vi "Start Module.vi"(7 "CfgManager":refnum<class "ConfigManager.lvclass">, 8 "error in (no error)":errorcluster, 9 "Owner":refnum<class "UniqueName.lvclass">, 10 "Module Name (empty: default)":string, 11 "Run as Singleton? (F)":bool) -> (0 "error out":errorcluster, 1 "Wait for Event Sync?":bool, 2 "Configurable Broadcast Events":T1, 3 "Module ID":i32)   [LabVIEW 2014, in "Configurable.lvlib"]
doc: "Launches the Module Main.vi.\n_____\nBased on Delacor QMH Project Template 4.0.0.47."
uses:
  Configurable.lvlib
  Broadcast Events--cluster.ctl
  Did Init Argument--cluster.ctl
  Status Updated Argument--cluster.ctl
  Error Reported Argument--cluster.ctl
  Stop Argument--cluster.ctl
  Get Module Execution Status Argument--cluster.ctl
  Module Configuration Argument--cluster.ctl
  ModuleConfiguration--Cluster.ctl
  <vilib>/LabVIEW Open Source/Configuration Manager/Manager/ConfigManager.lvclass
  <vilib>/LabVIEW Open Source Project/Unicity/UniqueName/UniqueNameClass/UniqueName.lvclass
  Module Running State--enum.ctl
  <vilib>/Delacor/Delacor QMH/Libraries/Cloneable Module Admin_class/Delacor_lib_QMH_Cloneable Module Admin.lvclass
  <vilib>/Delacor/Delacor QMH/Libraries/Cloneable Module Admin_class/Delacor_lib_QMH_Cloneable Module Admin.lvclass/Delacor_lib_QMH_Cloneable Module Admin.ctl
  <vilib>/Delacor/Delacor QMH/Libraries/Module Admin_class/Delacor_lib_QMH_Module Admin.lvclass/Delacor_lib_QMH_Module Admin.ctl
  <vilib>/Delacor/Delacor QMH/Libraries/Cloneable Module Admin_class/Delacor_lib_QMH_Set Module ID.vi
  <vilib>/Delacor/Delacor QMH/Libraries/Module Admin_class/Delacor_lib_QMH_Set External Launch.vi
  <vilib>/Utility/error.llb/Error Cluster From Error Code.vi
  <vilib>/ErrorRing/Error Ring.xnode
  Clone Registration/Clone Registration.lvlib
  <vilib>/LabVIEW Open Source/Configuration Manager/Cache/ConfigManager.Cache.lvclass
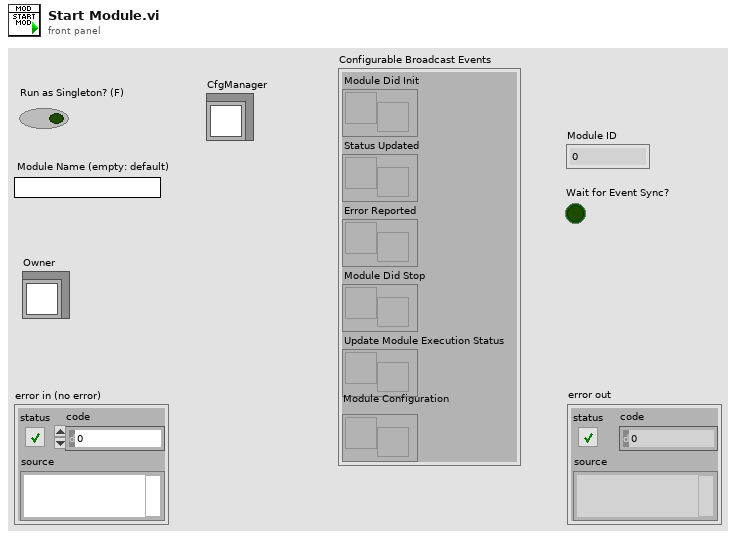
[diagram p1: front panel]
types:
  T1 = typedef "Configurable.lvlib/Broadcast Events--cluster.ctl" = cluster{"Module Did Init":refnum<user-event>, "Status Updated":refnum<user-event>, "Error Reported":refnum<user-event>, "Module Did Stop":refnum<user-event>, "Update Module Execution Status":refnum<user-event>, "Module Configuration":refnum<user-event>}
  T2 = typedef "Configurable.lvlib/Module Running State--enum.ctl" = enum16{"Not Running", "Running as Cloneable", "Running as Singleton"}
  T3 = enum32{"Bad", "Idle", "Run top level", "Running"}
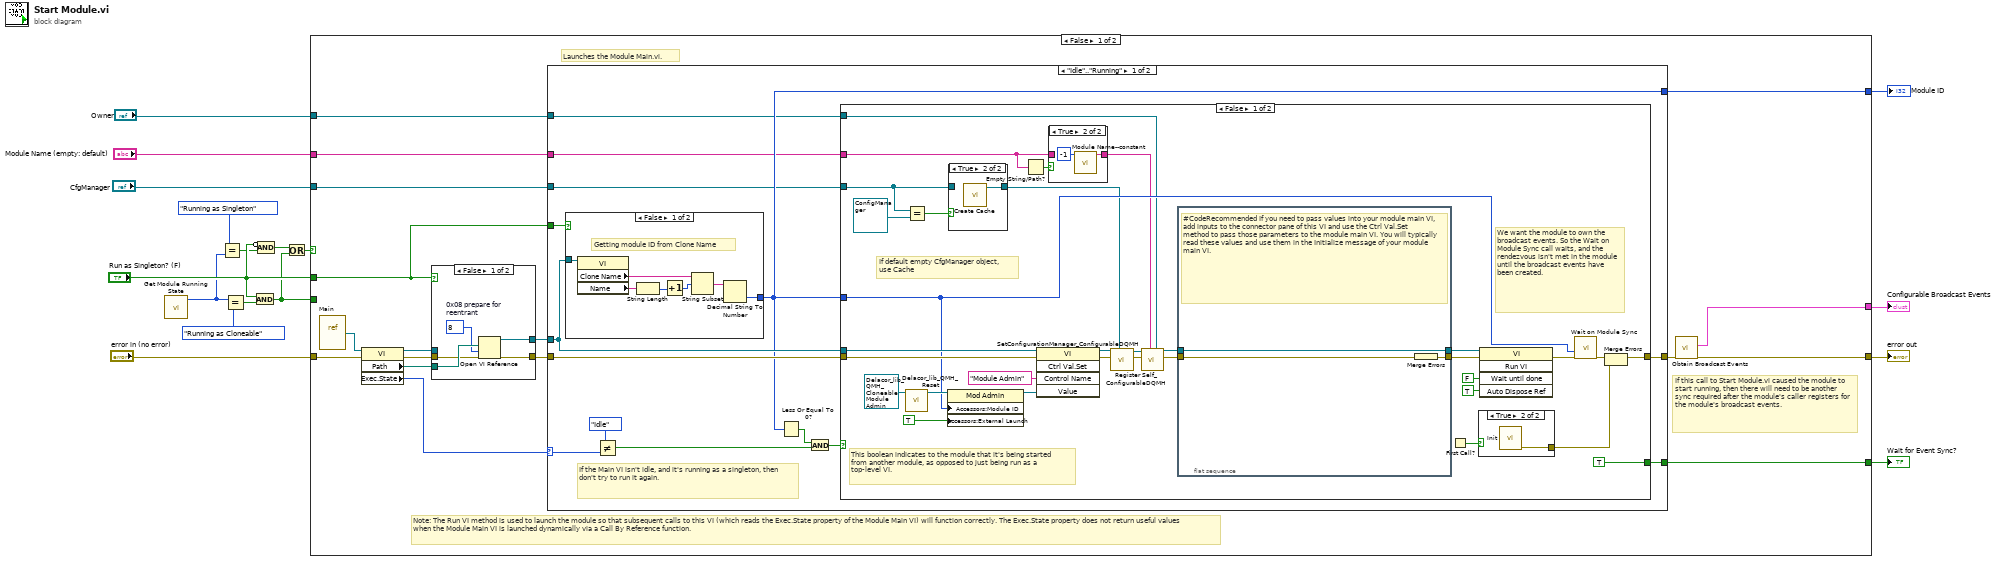
[diagram p0: block diagram]
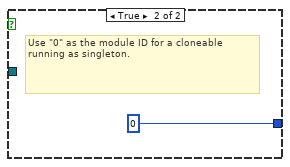
[diagram p3: hidden frame]
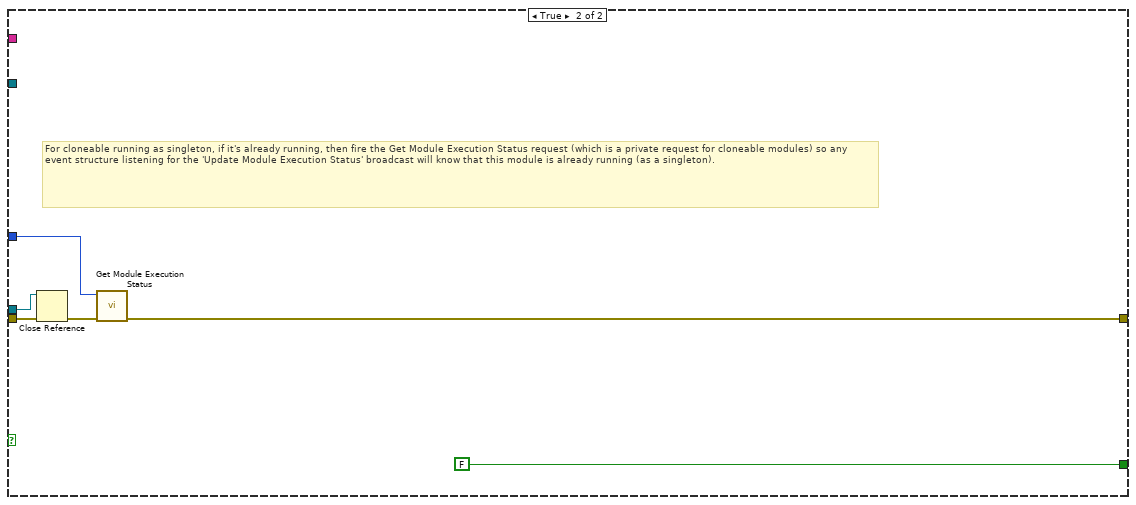
[diagram p7: hidden frame]
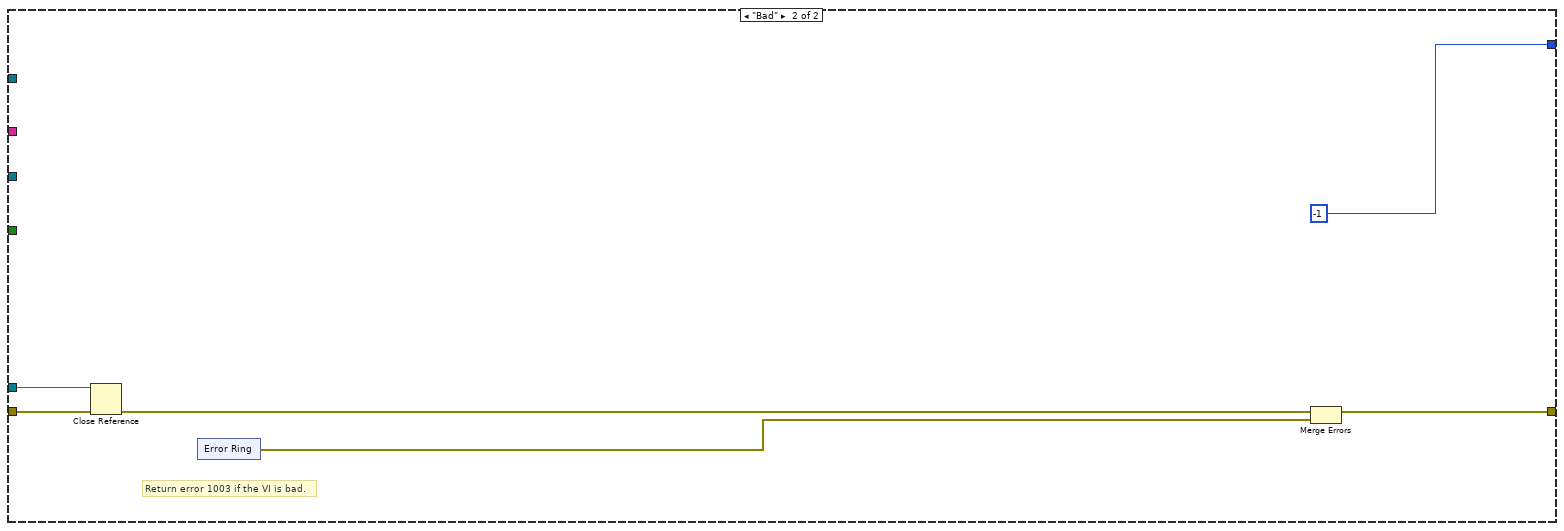
[diagram p8: hidden frame]
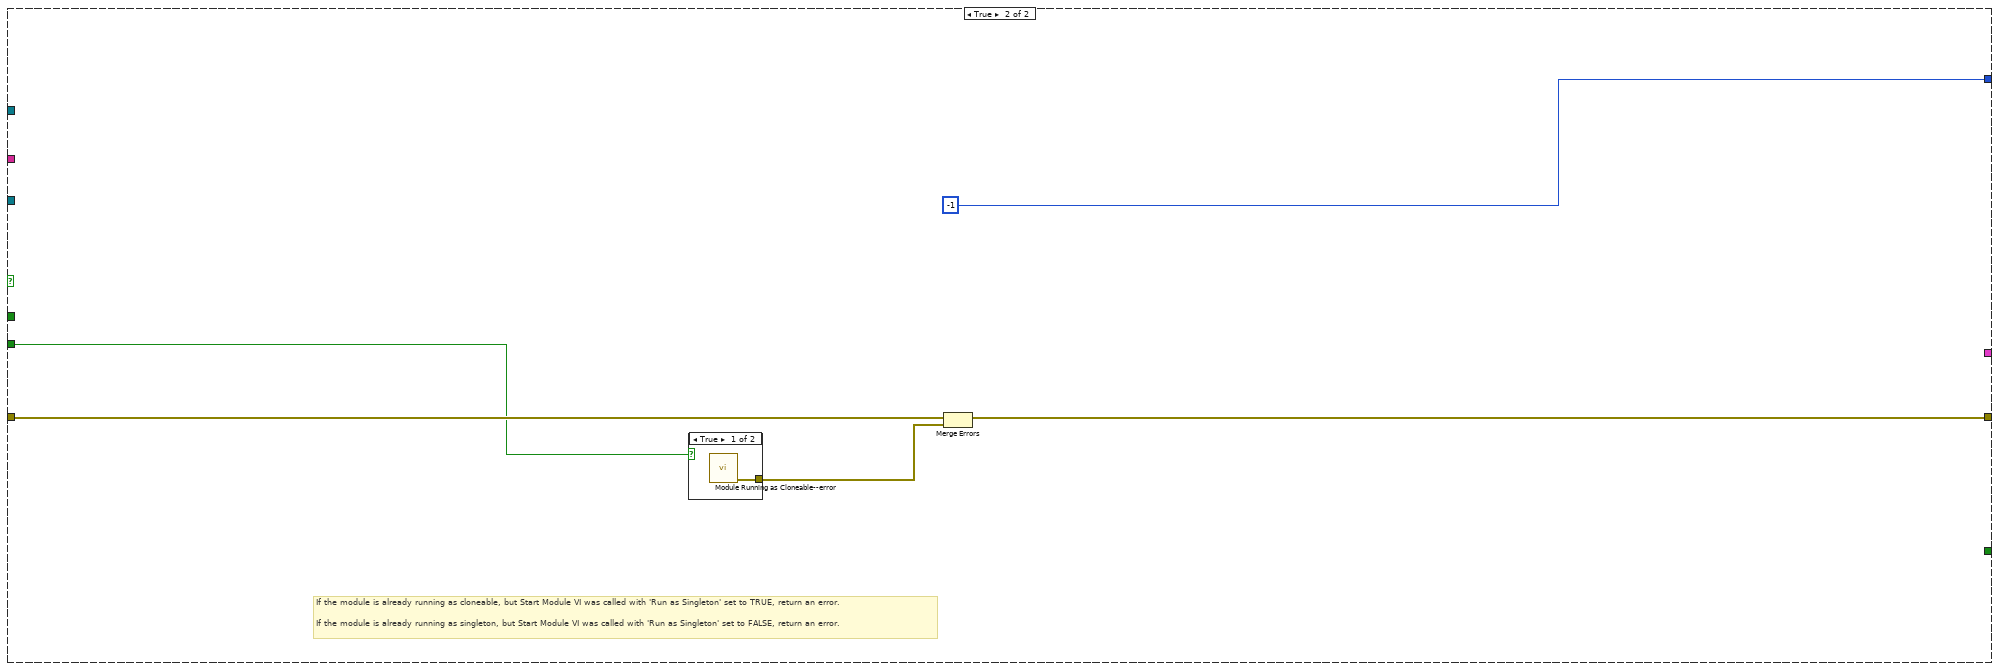
[diagram p9: hidden frame]
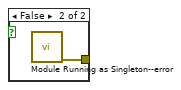
[diagram p10: hidden frame]
diagram:
  n1 = call "Get Module Running State.vi"() -> ("Module Running State"=w6:T2)  [unwired: 11 in]
  n2 = Equal?(x=Module_Running_State--enum."Running as Singleton", y=w6) -> (x = y?=w7:bool)
  n3 = Equal?(x=w6, y=Module_Running_State--enum."Running as Cloneable") -> (x = y?=w11:bool)
  n4 = And(x="Run as Singleton? (F)", y=w11) -> (x .and. y?=w4:bool)
  n5 = Compound Arithmetic op=AND(invert "Run as Singleton? (F)", w7) -> (w9:bool)
  n6 = Or(x=w9, y=w4) -> (x .or. y?=w10:bool)
  n7 = case shown="False" w10 {
    tunnel: "error in (no error)" -> [w34 w125]
    tunnel: [w32 w124] -> w16
    tunnel: [w31 _] -> w15
    tunnel: [w30 _] -> w14
    tunnel: [w26 -1] -> w13
    tunnel: "Run as Singleton? (F)" -> [w22 _]
    tunnel: w4 -> [_ w121]
    tunnel: "CfgManager" -> [w20 _]
    tunnel: "Module Name (empty: default)" -> [w19 _]
    tunnel: "Owner" -> [w18 _]
    frame False {
      # "Note: The Run VI method is used to launch the module so that subsequent calls to this VI (which reads the Exec.State property of the Module Main VI) will function correctly. The Exec.State property does not return useful values when the Module Main VI is launched dynamically via a Call By Reference function."
      # "If this call to Start Module.vi caused the module to start running, then there will need to be another sync required after the module's caller registers for the module's broadcast events."
      # "Launches the Module Main.vi."
      n8 = vi-ref "Main.vi"() -> (w25:refnum<vi>)
      n9 = property class="VI"(reference=w25, error in=w34) -> (reference out=w21:refnum<vi>, error out=w28:errorcluster, "Path"=w29:path, "Exec.State"=w23:T3)
      n10 = case shown="False" w22 {
        tunnel: w29 -> [w39 _]
        tunnel: w28 -> [w38 w41]
        tunnel: [w37 w41] -> w27
        tunnel: [w35 w40] -> w24
        tunnel: w21 -> [_ w40]
        frame False {
          w36 = 8  # 0x08 prepare for reentrant
          n11 = Open VI Reference(vi path=w39, options=w36, error in (no error)=w38) -> (vi reference=w35:refnum<vi>, error out=w37:errorcluster)  [unwired: 3 in]
        }
        frame True {
        }
      }
      n12 = case shown="\"Idle\"..\"Running\"" w23 {
        selector: w23 -> [w51 _]
        tunnel: w27 -> [w55 w116]
        tunnel: w24 -> [w53 w115]
        tunnel: [w52 w113] -> w33
        tunnel: [w54 _] -> w30
        tunnel: [w46 -1] -> w26
        tunnel: w22 -> [w45 _]
        tunnel: w20 -> [w44 _]
        tunnel: w19 -> [w43 _]
        tunnel: w18 -> [w42 _]
        frame "Idle".."Running" {
          # "If the Main VI isn't idle, and it's running as a singleton, then don't try to run it again."
          n13 = case shown="False" w45 {
            tunnel: w53 -> [w62 _]
            tunnel: [w56 0] -> w46
            frame False {
              # "Getting module ID from Clone Name"
              n14 = property class="VI"(reference=w62) -> ("Clone Name"=w59:string, "Name"=w58:string)  [unwired: 1 in, 2 out]
              n15 = String Length(string=w58) -> (length=w60:i32)
              n16 = Increment(x=w60) -> (x+1=w61:i32)
              n17 = String Subset ("Getting module ID from Clone Name")(string=w59, offset (0)=w61) -> (substring=w57:string)  [unwired: 1 in]
              n18 = Decimal String To Number(string=w57) -> (number=w56:i32)  [unwired: 2 in, 1 out]
            }
            frame True {
              # "Use \"0\" as the module ID for a cloneable running as singleton."
            }
          }
          n19 = Not Equal?(x=T3."Idle", y=w51) -> (x != y?=w49:bool)
          n20 = Less Or Equal To 0?(x=w46) -> (x <= 0?=w47:bool)
          n21 = And(x=w47, y=w49) -> (x .and. y?=w48:bool)
          n22 = case shown="False" w48 {
            tunnel: w55 -> [w95 w109]
            tunnel: [TRUE FALSE] -> w54
            tunnel: w53 -> [w88 w106]
            tunnel: [w86 w105] -> w52
            tunnel: w46 -> [w75 w108]
            tunnel: w44 -> [w76 _]
            tunnel: w43 -> [w73 _]
            tunnel: w42 -> [w65 _]
            frame False {
              # "If default empty CfgManager object,\nuse Cache"
              # "We want the module to own the broadcast events. So the Wait on Module Sync call waits, and the rendezvous isn't met in the module until the broadcast events have been created."
              # "This boolean indicates to the module that it's being started from another module, as opposed to just being run as a top-level VI."
              n23 = call-dynamic "Delacor_lib_QMH_Reset.vi"("Mod Admin in"=refnum<class "Delacor_lib_QMH_Cloneable Module Admin.lvclass"> refnum) -> ("Mod Admin out"=w84:refnum<class "Delacor_lib_QMH_Cloneable Module Admin.lvclass">)  [unwired: 9 in, 1 out]
              n24 = Equal?(x=w76, y=refnum<class "ConfigManager.lvclass"> refnum ("CfgManager")) -> (x = y?=w77:bool)
              n25 = property class="Mod Admin"(reference=w84, "Accessors:Module ID"=w75, "Accessors:External Launch"=TRUE) -> (reference out=w83:refnum<class "Delacor_lib_QMH_Cloneable Module Admin.lvclass">)  [unwired: 1 in, 1 out]
              n26 = case shown="True" w77 {
                tunnel: [w99 w100] -> w66
                tunnel: w76 -> [w99 _]
                frame False {
                }
                frame True {
                  n27 = call <vilib>:"Create Cache.vi"() -> ("ConfigManager.Cache"=w100:refnum<class "ConfigManager.Cache.lvclass">)  [unwired: 11 in]
                }
              }
              n28 = Empty String/Path?(string/path=w73) -> (empty?=w74:bool)
              n29 = invoke class="VI" method="Ctrl Val.Set"(reference=w88, error in=w95, "Control Name"="Module Admin", "Value"=w83) -> (reference out=w70:refnum<vi>, error out=w68:errorcluster)  [unwired: 1 in, 3 out]
              n30 = case shown="True" w74 {
                tunnel: w73 -> [w96 _]
                tunnel: [w96 w98] -> w64
                frame False {
                }
                frame True {
                  n31 = call "Module Name--constant.vi"("Module ID"=-1) -> ("Module Name"=w98:string)  [unwired: 10 in]
                }
              }
              n32 = call "SetConfigurationManager_ConfigurableDQMH.vi"("ConfigManager in"=w66, "error in (no error)"=w68, "vi reference in"=w70) -> ("error out"=w72:errorcluster, "vi reference out"=w71:refnum<vi>)  [unwired: 7 in]
              n33 = call "Register Self_ConfigurableDQMH.vi"("Ownwer"=w65, "Module Name"=w64, "error in (no error)"=w72, "vi reference in"=w71) -> ("error out"=w67:errorcluster, "vi reference out"=w69:refnum<vi>)  [unwired: 6 in]
              n34 = flat-sequence {
                tunnel: w69 -> [w102]
                tunnel: [w102] -> w80
                tunnel: w67 -> [w101]
                tunnel: [w103] -> w79
                frame #0 {
                  # "#CodeRecommended If you need to pass values into your module main VI, add inputs to the connector pane of this VI and use the Ctrl Val.Set method to pass those parameters to the module main VI. You will typically read these values and use them in the Initialize message of your module main VI."
                  n35 = Merge Errors(w101) -> (w103:errorcluster)
                }
              }
              n36 = First Call?() -> (First Call?: T/F=w87:bool)
              n37 = case shown="True" w87 {
                tunnel: [_ w104] -> w85
                frame False {
                }
                frame True {
                  n38 = call "Init.vi"() -> ("error out"=w104:errorcluster)  [unwired: 8 in, 3 out]
                }
              }
              n39 = invoke class="VI" method="Run VI"(reference=w80, error in=w79, "Wait until done"=FALSE ("Wait Until Done"), "Auto Dispose Ref"=TRUE ("Auto Dispose Reference")) -> (error out=w92:errorcluster)  [unwired: 1 in, 4 out]
              n40 = call "Wait on Module Sync.vi"("error in (no error)"=w92, "Module ID"=w75) -> ("error out"=w91:errorcluster)  [unwired: 9 in]
              n41 = Merge Errors(w91, w85) -> (w86:errorcluster)
            }
            frame True {
              # "For cloneable running as singleton, if it's already running, then fire the Get Module Execution Status request (which is a private request for cloneable modules) so any event structure listening for the 'Update Module Execution Status' broadcast will know that this module is already running (as a singleton)."
              n42 = Close Reference(reference=w106, error in (no error)=w109) -> (error out=w107:errorcluster)
              n43 = call "Get Module Execution Status.vi"("error in (no error)"=w107, "Module ID"=w108) -> ("error out"=w105:errorcluster)  [unwired: 9 in]
            }
          }
        }
        frame "Bad" {
          # "Return error 1003 if the VI is bad."
          n44 = Close Reference(reference=w115, error in (no error)=w116) -> (error out=w114:errorcluster)
          n45 = xnode "Error Ring"() -> ("error out"=w112:errorcluster)
          n46 = Merge Errors(w114, w112) -> (w113:errorcluster)
        }
      }
      n47 = call "Obtain Broadcast Events.vi"("error in (no error)"=w33) -> ("error out"=w32:errorcluster, "Configurable Broadcast Events"=w31:T1)  [unwired: 9 in]
    }
    frame True {
      # "If the module is already running as cloneable, but Start Module VI was called with 'Run as Singleton' set to TRUE, return an error.\n\nIf the module is already running as singleton, but Start Module VI was called with 'Run as Singleton' set to FALSE, return an error."
      n48 = case shown="True" w121 {
        tunnel: [w126 w127] -> w122
        frame True {
          n49 = call "Module Running as Cloneable--error.vi"() -> ("error out"=w126:errorcluster)  [unwired: 11 in]
        }
        frame False {
          n50 = call "Module Running as Singleton--error.vi"() -> ("error out"=w127:errorcluster)  [unwired: 11 in]
        }
      }
      n51 = Merge Errors(w125, w122) -> (w124:errorcluster)
    }
  }
  "error out" <- w16
  "Configurable Broadcast Events" <- w15
  "Wait for Event Sync?" <- w14
  "Module ID" <- w13
